vi "Configure Offset and Limits (Spectrum Emission Mask - Frequency and Offset Side).vi"(0 "VISA resource name":refnum<visa-resource-name>, 1 "Manual Start Frequency List":dbl[](array[numeric])=[2515000.0, 2515000.0, 2515000.0, 2515000.0, 2515000.0, 2515000.0] format="%#.6g", 5 "Device Mode (1: BTS)":i32(ring)=1 items=["BTS"=1, "MS"=2], 7 "Offset Side List":i32[](array[ring])=[0, 0, 0, 0, 0, 0] items=["Both", "Negative", "Positive"], 9 "Auto Start Frequency List":bool[](array[boolean])=[TRUE, TRUE, TRUE, TRUE, TRUE, TRUE], 11 "error in (no error)":errorcluster, 12 "Stop Frequency List":dbl[](array[numeric])=[2715000.0, 2715000.0, 2715000.0, 2715000.0, 2715000.0, 2715000.0] format="%#.6g") -> (4 "VISA resource name out":refnum<visa-resource-name>, 15 "error out":errorcluster)   [LabVIEW 2018, in "Agilent MXA Series.lvlib"]
doc: "Configures the frequency and offset side settings under the offsets and limits for Spectrum Emission Mask measurement type."
uses:
  Agilent MXA Series.lvlib
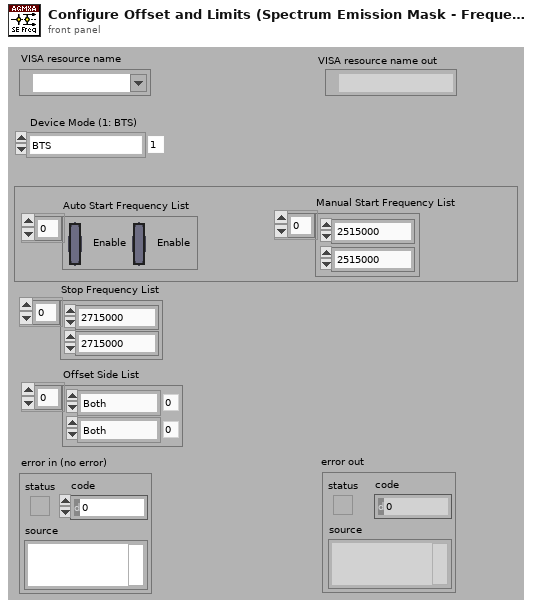
[diagram p1: front panel]
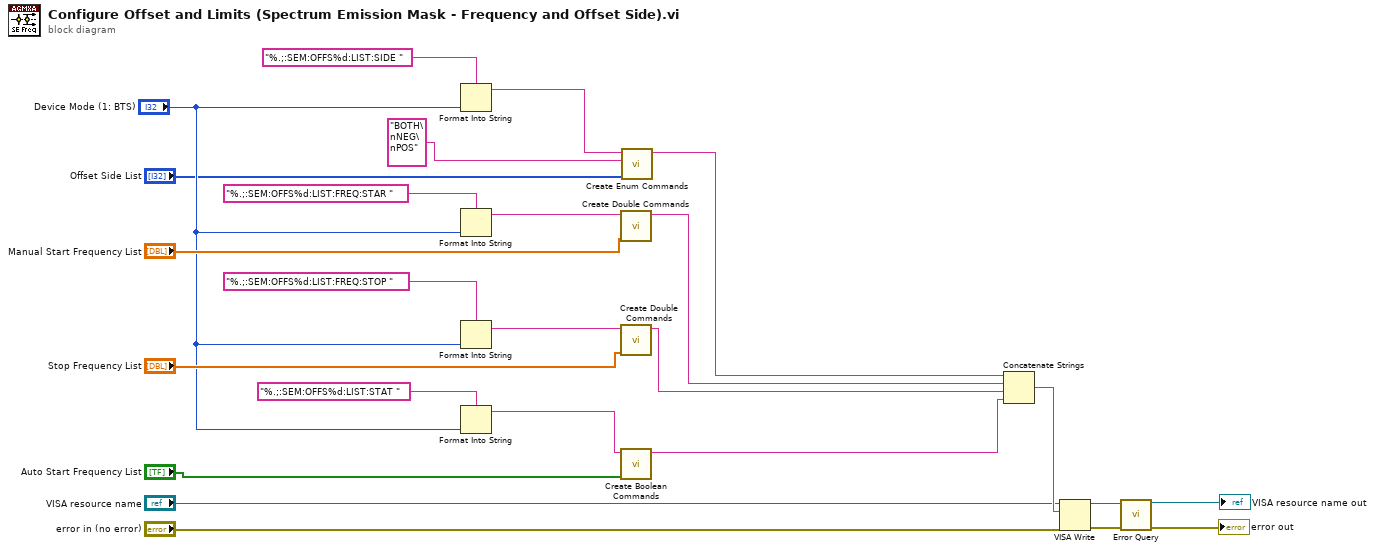
[diagram p0: block diagram]
diagram:
  n1 = Format Into String(format string="%.;:SEM:OFFS%d:LIST:SIDE ", "Device Mode (1: BTS)") -> (resulting string=w2:string)  [unwired: 2 in, 1 out]
  n2 = Format Into String(format string="%.;:SEM:OFFS%d:LIST:FREQ:STAR ", "Device Mode (1: BTS)") -> (resulting string=w21:string)  [unwired: 2 in, 1 out]
  n3 = Format Into String(format string="%.;:SEM:OFFS%d:LIST:FREQ:STOP ", "Device Mode (1: BTS)") -> (resulting string=w17:string)  [unwired: 2 in, 1 out]
  n4 = Format Into String(format string="%.;:SEM:OFFS%d:LIST:STAT ", "Device Mode (1: BTS)") -> (resulting string=w23:string)  [unwired: 2 in, 1 out]
  n5 = call "Create Double Commands.vi"("Double Values"="Manual Start Frequency List", "Commands"=w21) -> ("Result"=w14:string)  [unwired: 9 in]
  n6 = call "Create Double Commands.vi"("Double Values"="Stop Frequency List", "Commands"=w17) -> ("Result"=w13:string)  [unwired: 9 in]
  n7 = call "Create Boolean Commands.vi"("Boolean States"="Auto Start Frequency List", "Command"=w23) -> ("Result String"=w12:string)  [unwired: 9 in]
  n8 = call "Create Enum Commands.vi"("Enum Values"="Offset Side List", "Multi-line Text"="BOTH\nNEG\nPOS" ("multi-line string"), "Commands"=w2) -> ("Result"=w1:string)  [unwired: 8 in]
  n9 = Concatenate Strings(w1, w14, w13, w12) -> (w11:string)
  n10 = VISA Write(VISA resource name="VISA resource name", write buffer=w11, error in (no error)="error in (no error)") -> (VISA resource name out=w7:refnum<visa-resource-name>, error out=w8:errorcluster)  [unwired: 1 out]
  n11 = call "Error Query.vi"("error in (no error)"=w8, "VISA resource name"=w7) -> ("error out"=→"error out":errorcluster, "VISA resource name out"=→"VISA resource name out":refnum<visa-resource-name>)  [unwired: 6 in, 2 out]
